vi "Initialize Counter Task.vi"(8 "error in (no error)":errorcluster, 11 "BNT_DAQmx-MCSV in":refnum<class "BNT_DAQmx-MCSV.lvclass">) -> (0 "error out":errorcluster, 3 "Counter DAQmx Task":refnum<k21>)   [LabVIEW 2017, in "BNT_DAQmx.lvlib" / "BNT_DAQmx-MCSV.lvclass"]
doc: "Initialize DAQmx Counter task.\n\n<b>Default Implementation:</b> Count Edges\n\nThis dynamic dispatch VI can be overritten by derived classes to implement other counter tasks."
uses:
  BNT_DAQmx-MCSV.lvclass
  C:/User/Brand/LVP/Acc/VacuumHeating/Packages/CSPP_Core/Actors/CSPP_BaseActor/CSPP_BaseActor.lvclass
  CSPP_Core/Actors/CSPP_BaseActor/CSPP_BaseActor.lvclass/CSPP_BaseActor.ctl
  BNT_DAQmx-MCSV.lvclass/BNT_DAQmx-MCSV.ctl
  <vilib>/DAQmx/create/channels.llb/DAQmx Create Channel (CI-Count Edges).vi
  CSPP_Core/Actors/CSPP_BaseActor/CSPP_BaseActor.lvclass
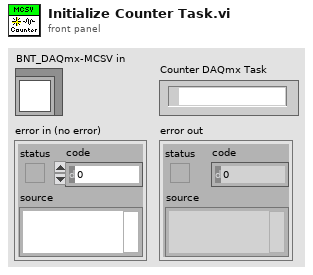
[diagram p1: front panel]
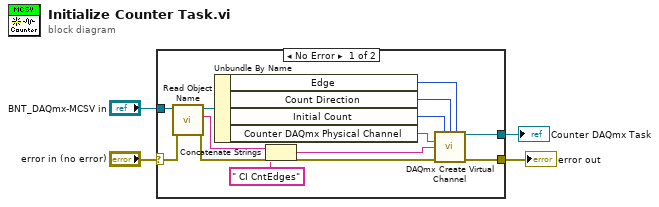
[diagram p0: block diagram]
diagram:
  n1 = case shown="No Error" "error in (no error)" {
    selector: "error in (no error)" -> [w9 w18]
    tunnel: [w15 w18] -> w3
    tunnel: "BNT_DAQmx-MCSV in" -> [w11 _]
    tunnel: [w14 _] -> w1
    frame No Error {
      n2 = call "Read Object Name.vi"("error in (no error)"=w9, "CSPP_BaseActor in"=w11) -> ("error out"=w8:errorcluster, "Object Name"=w7:string, "CSPP_BaseActor out"=w10:refnum<class "BNT_DAQmx-MCSV.lvclass">)  [unwired: 7 in]
      n3 = Unbundle By Name(w10) -> ("Edge"=w17:i32, "Count Direction"=w13:i32, "Initial Count"=w12:u32, "Counter DAQmx Physical Channel"=w16:tag)
      n4 = Concatenate Strings(w7, " CI CntEdges" ("string")) -> (w6:string)
      n5 = call-poly <vilib>:"DAQmx Create Virtual Channel.vi"("initial count"=w12, "count direction"=w13, "edge"=w17, "counter"=w16, "name to assign"=w6, "error in"=w8) -> ("task out"=w14:refnum<k21>, "error out"=w15:errorcluster)  [unwired: 8 in]
    }
    frame Error {
    }
  }
  "error out" <- w3
  "Counter DAQmx Task" <- w1
